vi "Tarea 16.vi"() -> ()   [LabVIEW 2019]
uses:
  Student Material/Student Material/Module 4/Exercises 16/Solutions/CLD 16 state enum.ctl
  Student Material/Student Material/Module 4/Exercises 16/Controls/CLD 16 Status Panel.ctl
  Student Material/Student Material/Module 4/Exercises 16/Controls/CLD 16 Control Panel.ctl
  Student Material/Student Material/Module 4/Exercises 16/Solutions/CLD 16 Data Cluster.ctl
panel:
  out "Error Out":errorcluster
  in  "Error In":errorcluster
  in  "Control Panel Line Two":T1 {"Tons of Peanuts" scale=0.0..10.0}
  in  "Control Panel Line One":T1 {"Tons of Peanuts" scale=0.0..10.0}
  out "Process Control":T2 {"Process Value" format="%#.3g"}
  out "Line One Active":bool
  out "Line Two Active":bool
  in  "Stop Button":bool
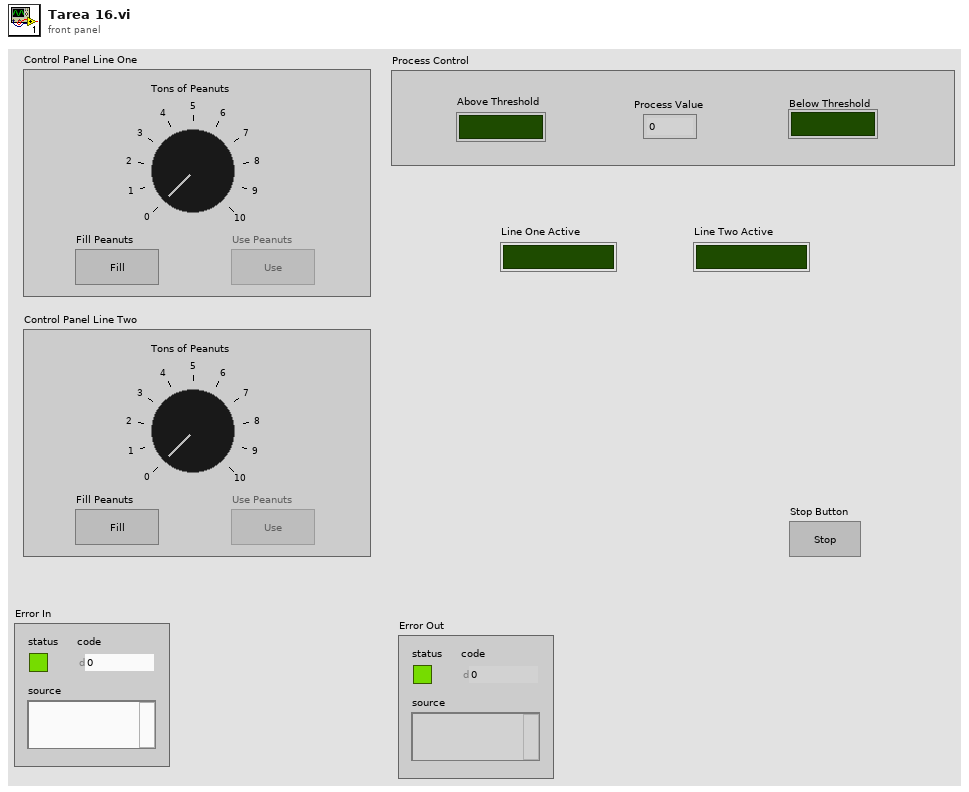
[diagram p1: front panel]
types:
  T1 = typedef "CLD 16 Control Panel.ctl" = cluster{"Tons of Peanuts":i8, "Fill Peanuts":bool, "Use Peanuts":bool}
  T2 = typedef "CLD 16 Status Panel.ctl" = cluster{"Above Threshold":bool, "Below Threshold":bool, "Process Value":dbl}
  T3 = typedef "CLD 16 Data Cluster.ctl" = cluster{"Control Panel Array":T1[], "Status Panel":T2, "Line One":bool, "Line Two":bool, "Stop Button":bool}
  T4 = typedef "CLD 16 state enum.ctl" = enum16{"initialize", "use", "idle"}
  T5 = enum8{"Enabled", "Disabled", "Disabled and Grayed Out"}
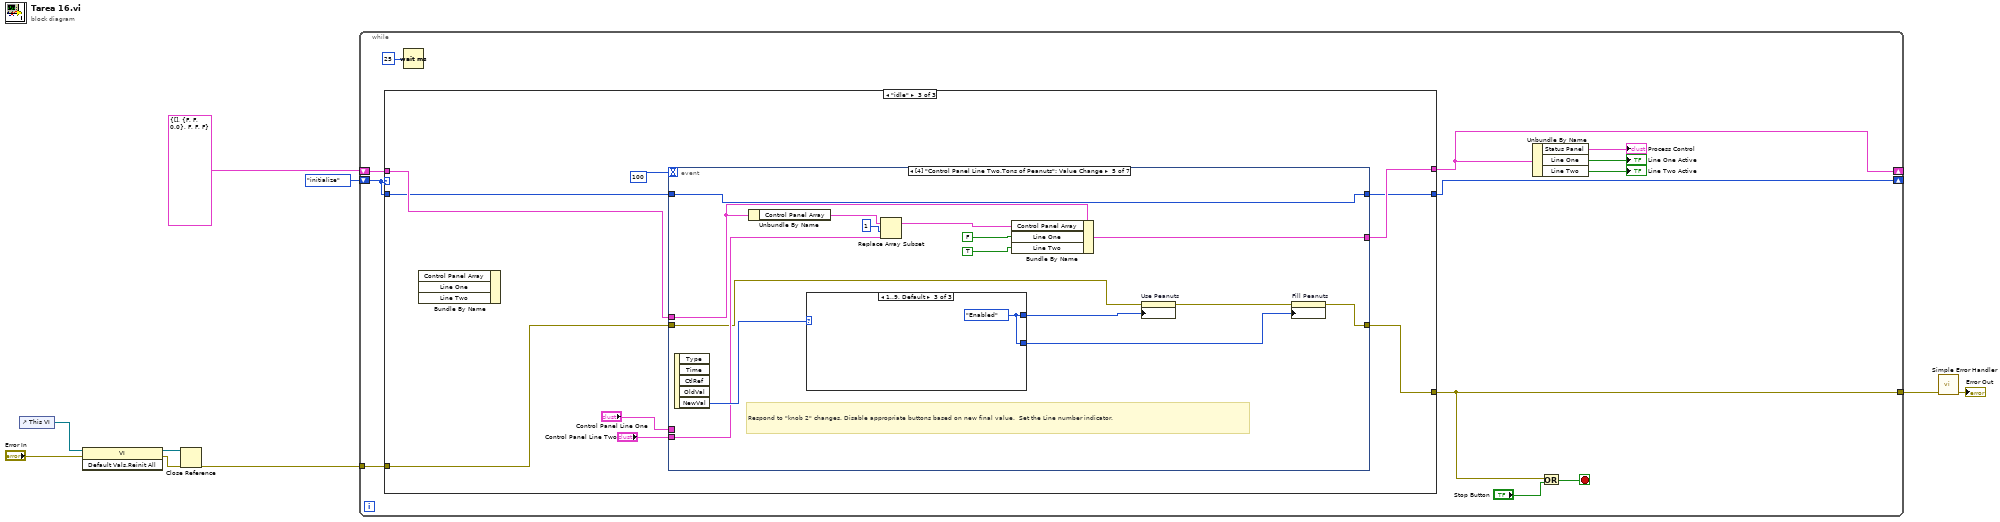
[diagram p0: block diagram]
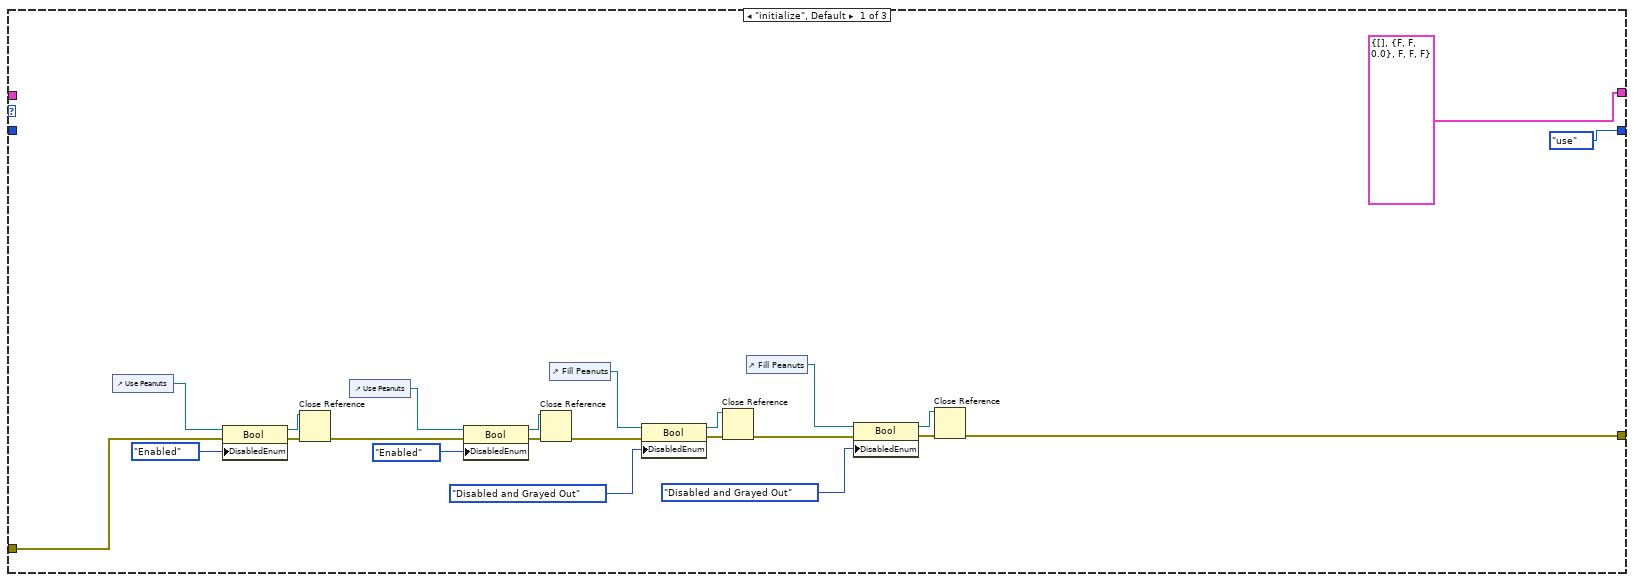
[diagram p2: hidden frame]
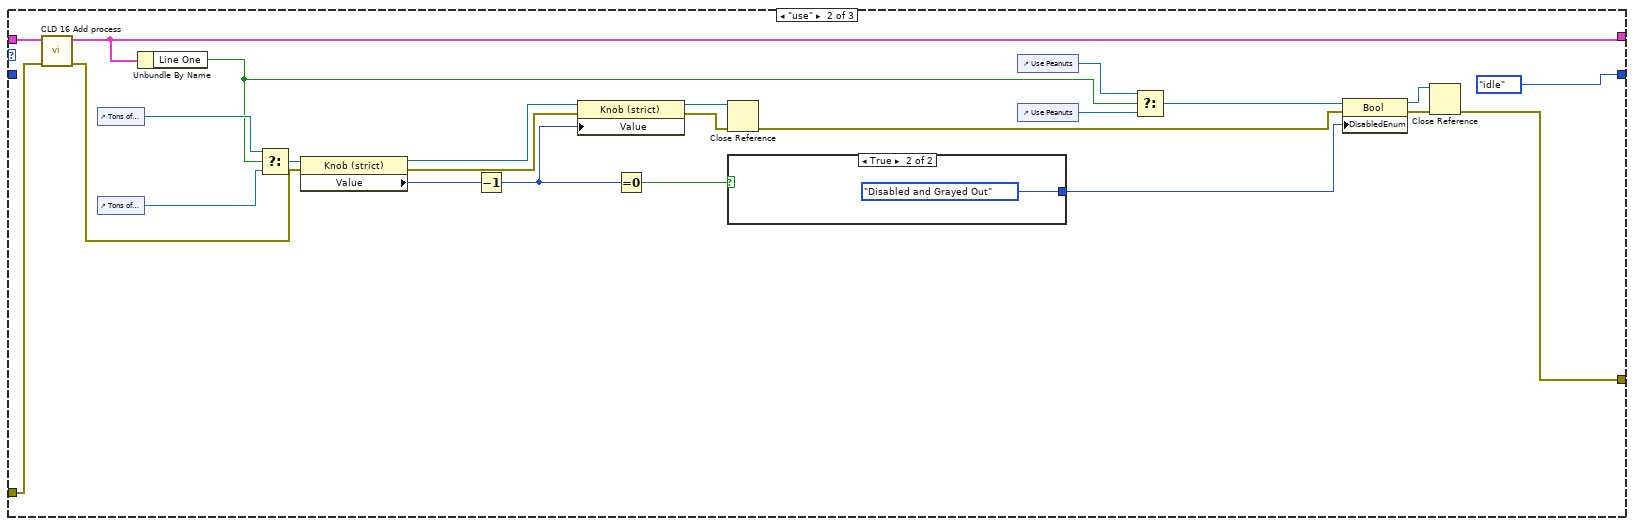
[diagram p3: hidden frame]
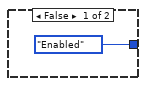
[diagram p4: hidden frame]
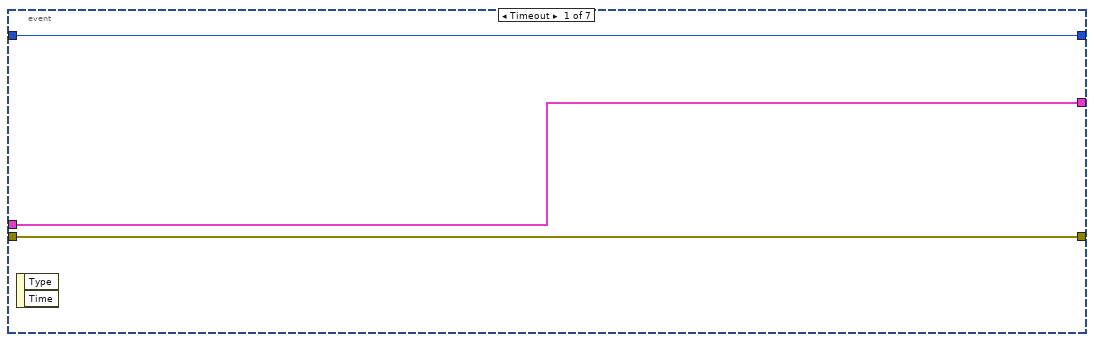
[diagram p5: hidden frame]
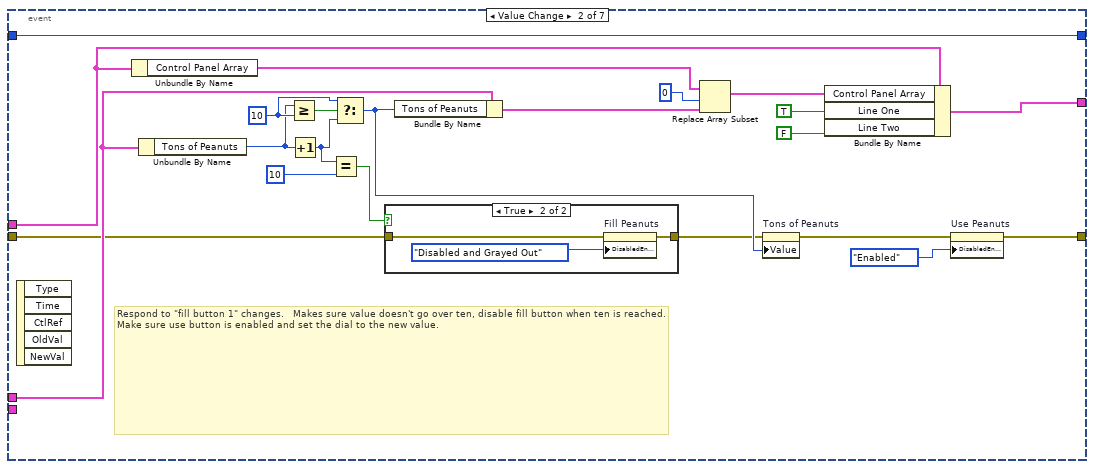
[diagram p6: hidden frame]
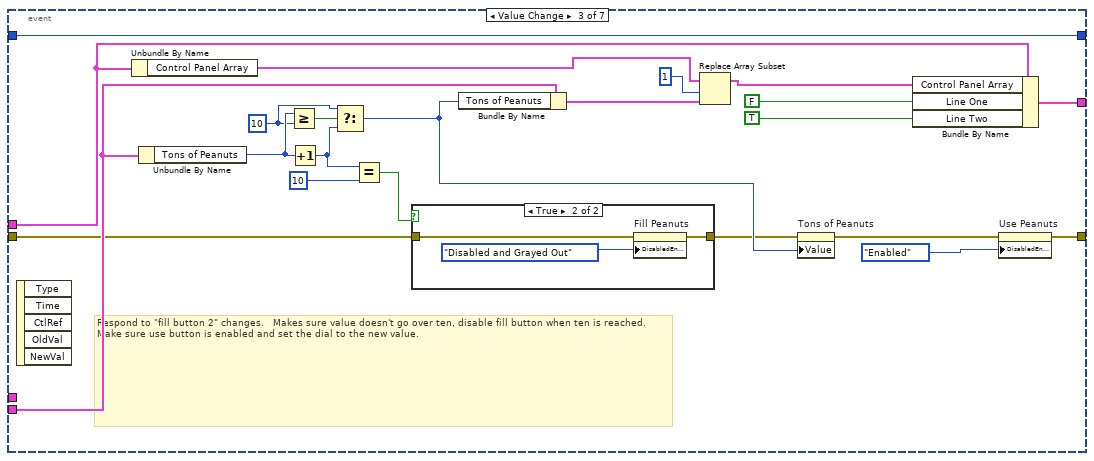
[diagram p8: hidden frame]
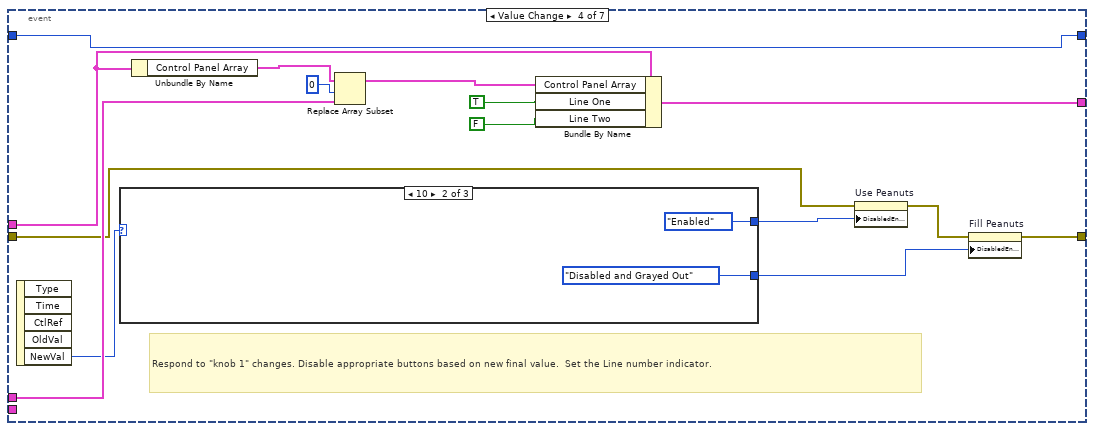
[diagram p10: hidden frame]
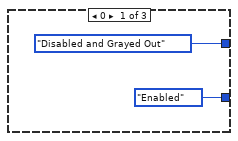
[diagram p11: hidden frame]
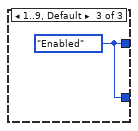
[diagram p12: hidden frame]
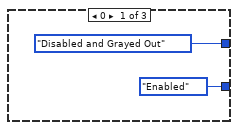
[diagram p13: hidden frame]
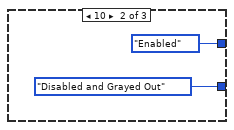
[diagram p14: hidden frame]
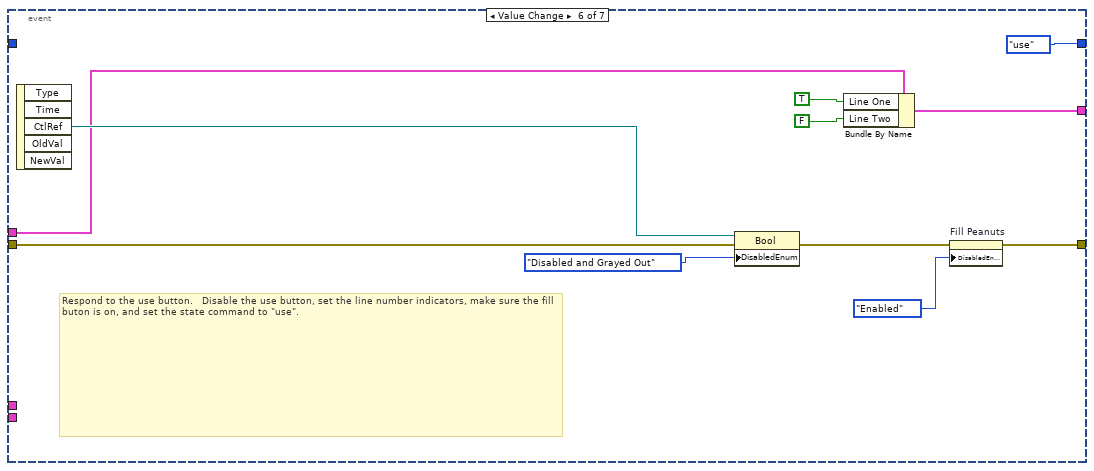
[diagram p15: hidden frame]
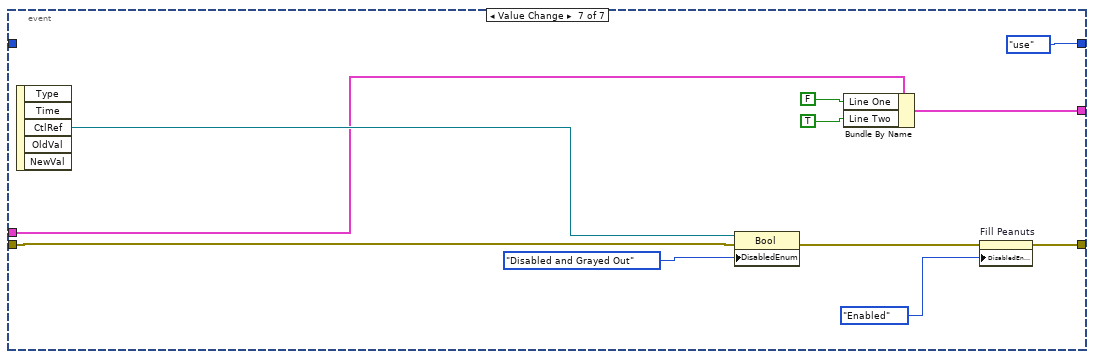
[diagram p16: hidden frame]
diagram:
  n1 = control-ref of="This VI"() -> (w4:refnum<vi>)
  n2 = invoke class="VI" method="Default Vals.Reinit All"(reference=w4, error in="Error In") -> (reference out=w2:refnum<vi>, error out=w5:errorcluster)  [unwired: 1 in, 1 out]
  n3 = Close Reference(reference=w2, error in (no error)=w5) -> (error out=w3:errorcluster)
  n4 = while {
    shift-right: [w20] -> _
    shift-left: CLD_16_state_enum."initialize" ("CLD 16 States") -> [w21]
    shift-right: [w15] -> _
    shift-left: T3 {"Control Panel Array"=[], "Status Panel"={"Above Threshold"=FALSE, "Below Threshold"=FALSE, "Process Value"=0.0}, "Line One"=FALSE, "Line Two"=FALSE, "Stop Button"=FALSE} ("Cluster") -> [w19]
    tunnel: [w10] -> w8
    tunnel: w3 -> [w18]
    stop <- w17 stop-if-true
    n5 = case shown="\"idle\"" w21 {
      tunnel: [CLD_16_state_enum."use" ("CLD 16 States") CLD_16_state_enum."idle" ("CLD 16 States") w74] -> w20
      tunnel: w21 -> [_ _ w75]
      tunnel: w19 -> [_ w68 w79]
      tunnel: [T3 {"Control Panel Array"=[], "Status Panel"={"Above Threshold"=FALSE, "Below Threshold"=FALSE, "Process Value"=0.0}, "Line One"=FALSE, "Line Two"=FALSE, "Stop Button"=FALSE} ("Cluster") w66 w78] -> w15
      tunnel: [w22 w47 w71] -> w10
      tunnel: w18 -> [w29 w46 w72]
      frame "initialize", Default {
        n6 = control-ref of="Use Peanuts"() -> (w30:refnum<vi>)
        n7 = property class="Bool"(reference=w30, error in=w29, "DisabledEnum"=T5."Enabled" ("Disabled")) -> (reference out=w40:refnum<vi>, error out=w42:errorcluster)
        n8 = Close Reference(reference=w40, error in (no error)=w42) -> (error out=w28:errorcluster)
        n9 = control-ref of="Use Peanuts"() -> (w27:refnum<vi>)
        n10 = property class="Bool"(reference=w27, error in=w28, "DisabledEnum"=T5."Enabled" ("Disabled")) -> (reference out=w37:refnum<vi>, error out=w39:errorcluster)
        n11 = Close Reference(reference=w37, error in (no error)=w39) -> (error out=w26:errorcluster)
        n12 = control-ref of="Fill Peanuts"() -> (w25:refnum<vi>)
        n13 = property class="Bool"(reference=w25, error in=w26, "DisabledEnum"=T5."Disabled and Grayed Out" ("Disabled")) -> (reference out=w35:refnum<vi>, error out=w36:errorcluster)
        n14 = Close Reference(reference=w35, error in (no error)=w36) -> (error out=w24:errorcluster)
        n15 = control-ref of="Fill Peanuts"() -> (w23:refnum<vi>)
        n16 = property class="Bool"(reference=w23, error in=w24, "DisabledEnum"=T5."Disabled and Grayed Out" ("Disabled")) -> (reference out=w32:refnum<vi>, error out=w33:errorcluster)
        n17 = Close Reference(reference=w32, error in (no error)=w33) -> (error out=w22:errorcluster)
      }
      frame "use" {
        n18 = call "CLD 16 Add process.vi"("error in (no error)"=w46, "Cluster in"=w68) -> ("error out"=w45:errorcluster, "Cluster out"=w66:T3)  [unwired: 8 in]
        n19 = control-ref of="Tons of Peanuts"() -> (w58:refnum<vi>)
        n20 = control-ref of="Tons of Peanuts"() -> (w59:refnum<vi>)
        n21 = Unbundle By Name(w66) -> ("Line One"=w57:bool)
        n22 = Select(t=w58, s=w57, f=w59) -> (s? t:f=w55:refnum<vi>)
        n23 = property class="Knob (strict)"(reference=w55, error in=w45) -> (reference out=w54:refnum<vi>, error out=w49:errorcluster, "Value"=w56:i8)
        n24 = Decrement(x=w56) -> (x-1=w51:i8)
        n25 = property class="Knob (strict)"(reference=w54, error in=w49, "Value"=w51) -> (reference out=w52:refnum<vi>, error out=w53:errorcluster)
        n26 = Equal To 0?(x=w51) -> (x = 0?=w50:bool)
        n27 = Close Reference(reference=w52, error in (no error)=w53) -> (error out=w48:errorcluster)
        n28 = case shown="True" w50 {
          tunnel: [T5."Enabled" ("Disabled") T5."Disabled and Grayed Out" ("Disabled")] -> w63
          frame False {
          }
          frame True {
          }
        }
        n29 = control-ref of="Use Peanuts"() -> (w65:refnum<vi>)
        n30 = control-ref of="Use Peanuts"() -> (w62:refnum<vi>)
        n31 = Select(t=w65, s=w57, f=w62) -> (s? t:f=w64:refnum<vi>)
        n32 = property class="Bool"(reference=w64, error in=w48, "DisabledEnum"=w63) -> (reference out=w60:refnum<vi>, error out=w61:errorcluster)
        n33 = Close Reference(reference=w60, error in (no error)=w61) -> (error out=w47:errorcluster)
      }
      frame "idle" {
        n34 = Bundle By Name() -> ()  [unwired: 4 in, 1 out]
        n35 = event shown="[4] \"Control Panel Line Two.Tons of Peanuts\": Value Change" {
          selector: _ -> [_ _ _ _ _ _ _]
          dyn-events: _ -> [_ _ _ _ _ _ _]
          timeout: 100 -> [_ _ _ _ _ _ _]
          tunnel: w79 -> [w81 w103 w129 w148 w168 w180 w191]
          tunnel: [w81 w104 w130 w149 w169 w179 w190] -> w78
          tunnel: "Control Panel Line One" -> [_ w96 _ w141 _ _ _]
          tunnel: [w82 w99 w125 w144 w164 CLD_16_state_enum."use" ("CLD 16 States") CLD_16_state_enum."use" ("CLD 16 States")] -> w74
          tunnel: w75 -> [w82 w99 w125 w144 w164 _ _]
          tunnel: "Control Panel Line Two" -> [_ _ w116 _ w159 _ _]
          tunnel: w72 -> [w80 w91 w115 w138 w158 w178 w189]
          tunnel: [w80 w89 w113 w136 w156 w176 w187] -> w71
          event Timeout {
            n36 = event-data() -> ()  [unwired: 1 in, 2 out]
          }
          event Value Change {
            w92 = i8 10 ("x")
            # "Respond to \"fill button 1\" changes.   Makes sure value doesn't go over ten, disable fill button when ten is reached. Make sure use button is enabled and set the dial to the new value."
            n37 = event-data() -> ()  [unwired: 1 in, 5 out]
            n38 = Unbundle By Name(w103) -> ("Control Panel Array"=w102:T1[])
            n39 = Unbundle By Name(w96) -> ("Tons of Peanuts"=w84:i8)
            n40 = Greater Or Equal?(x=w84, y=w92) -> (x >= y?=w87:bool)
            n41 = Increment(x=w84) -> (x+1=w83:i8)
            n42 = Equal?(x=w83, y=i8 10 ("x")) -> (x = y?=w85:bool)
            n43 = Select(t=w92, s=w87, f=w83) -> (s? t:f=w93:i8)
            n44 = case shown="True" w85 {
              tunnel: w91 -> [w105 w108]
              tunnel: [w105 w107] -> w88
              frame False {
              }
              frame True {
                n45 = property on="Fill Peanuts" class="Bool"(error in=w108, "DisabledEnum"=T5."Disabled and Grayed Out" ("Disabled")) -> (error out=w107:errorcluster)  [unwired: 1 in, 1 out]
              }
            }
            n46 = Bundle By Name(cluster=w96, "Tons of Peanuts"=w93) -> (w95:T1)
            n47 = Replace Array Subset(array=w102, new element=w95, index=0) -> (w100:T1[])
            n48 = property on="Tons of Peanuts" class="Knob (strict)"(error in=w88, "Value"=w93) -> (error out=w90:errorcluster)  [unwired: 1 in, 1 out]
            n49 = Bundle By Name(cluster=w103, "Control Panel Array"=w100, "Line One"=TRUE, "Line Two"=FALSE ("Line One")) -> (w104:T3)
            n50 = property on="Use Peanuts" class="Bool"(error in=w90, "DisabledEnum"=T5."Enabled" ("Disabled")) -> (error out=w89:errorcluster)  [unwired: 1 in, 1 out]
          }
          event Value Change {
            w117 = i8 10 ("x")
            # "Respond to \"fill button 2\" changes.   Makes sure value doesn't go over ten, disable fill button when ten is reached. Make sure use button is enabled and set the dial to the new value."
            n51 = event-data() -> ()  [unwired: 1 in, 5 out]
            n52 = Unbundle By Name(w129) -> ("Control Panel Array"=w128:T1[])
            n53 = Unbundle By Name(w116) -> ("Tons of Peanuts"=w118:i8)
            n54 = Greater Or Equal?(x=w118, y=w117) -> (x >= y?=w120:bool)
            n55 = Increment(x=w118) -> (x+1=w111:i8)
            n56 = Select(t=w117, s=w120, f=w111) -> (s? t:f=w119:i8)
            n57 = Equal?(x=w111, y=i8 10 ("x")) -> (x = y?=w109:bool)
            n58 = case shown="True" w109 {
              tunnel: w115 -> [w131 w134]
              tunnel: [w131 w133] -> w110
              frame False {
              }
              frame True {
                n59 = property on="Fill Peanuts" class="Bool"(error in=w134, "DisabledEnum"=T5."Disabled and Grayed Out" ("Disabled")) -> (error out=w133:errorcluster)  [unwired: 1 in, 1 out]
              }
            }
            n60 = Bundle By Name(cluster=w116, "Tons of Peanuts"=w119) -> (w122:T1)
            n61 = Replace Array Subset(array=w128, new element=w122, index=1) -> (w126:T1[])
            n62 = property on="Tons of Peanuts" class="Knob (strict)"(error in=w110, "Value"=w119) -> (error out=w114:errorcluster)  [unwired: 1 in, 1 out]
            n63 = Bundle By Name(cluster=w129, "Control Panel Array"=w126, "Line One"=FALSE, "Line Two"=TRUE ("Line One")) -> (w130:T3)
            n64 = property on="Use Peanuts" class="Bool"(error in=w114, "DisabledEnum"=T5."Enabled" ("Disabled")) -> (error out=w113:errorcluster)  [unwired: 1 in, 1 out]
          }
          event Value Change {
            # "Respond to \"knob 1\" changes. Disable appropriate buttons based on new final value.  Set the Line number indicator."
            n65 = event-data() -> ("NewVal"=w139:i8)  [unwired: 1 in, 4 out]
            n66 = case shown="10" w139 {
              tunnel: [T5."Disabled and Grayed Out" ("Disabled") T5."Enabled" ("Disabled") w154] -> w140
              tunnel: [T5."Enabled" ("Disabled") T5."Disabled and Grayed Out" ("Disabled") w154] -> w135
              frame 0 {
              }
              frame 10 {
              }
              frame 1..9, Default {
                w154 = T5."Enabled" ("Disabled")
              }
            }
            n67 = Unbundle By Name(w148) -> ("Control Panel Array"=w147:T1[])
            n68 = Replace Array Subset(array=w147, new element=w141, index=0) -> (w145:T1[])
            n69 = Bundle By Name(cluster=w148, "Control Panel Array"=w145, "Line One"=TRUE, "Line Two"=FALSE ("Line One")) -> (w149:T3)
            n70 = property on="Use Peanuts" class="Bool"(error in=w138, "DisabledEnum"=w140) -> (error out=w137:errorcluster)  [unwired: 1 in, 1 out]
            n71 = property on="Fill Peanuts" class="Bool"(error in=w137, "DisabledEnum"=w135) -> (error out=w136:errorcluster)  [unwired: 1 in, 1 out]
          }
          event Value Change {
            # "Respond to \"knob 2\" changes. Disable appropriate buttons based on new final value.  Set the Line number indicator."
            n72 = event-data() -> ("NewVal"=w160:i8)  [unwired: 1 in, 4 out]
            n73 = Unbundle By Name(w168) -> ("Control Panel Array"=w167:T1[])
            n74 = case shown="1..9, Default" w160 {
              tunnel: [T5."Disabled and Grayed Out" ("Disabled") T5."Enabled" ("Disabled") w174] -> w161
              tunnel: [T5."Enabled" ("Disabled") T5."Disabled and Grayed Out" ("Disabled") w174] -> w155
              frame 0 {
              }
              frame 10 {
              }
              frame 1..9, Default {
                w174 = T5."Enabled" ("Disabled")
              }
            }
            n75 = Replace Array Subset(array=w167, new element=w159, index=1) -> (w165:T1[])
            n76 = Bundle By Name(cluster=w168, "Control Panel Array"=w165, "Line One"=FALSE, "Line Two"=TRUE ("Line One")) -> (w169:T3)
            n77 = property on="Use Peanuts" class="Bool"(error in=w158, "DisabledEnum"=w161) -> (error out=w157:errorcluster)  [unwired: 1 in, 1 out]
            n78 = property on="Fill Peanuts" class="Bool"(error in=w157, "DisabledEnum"=w155) -> (error out=w156:errorcluster)  [unwired: 1 in, 1 out]
          }
          event Value Change {
            # "Respond to the use button.   Disable the use button, set the line number indicators, make sure the fill buton is on, and set the state command to \"use\"."
            n79 = event-data() -> ("CtlRef"=w184:refnum<vi>)  [unwired: 1 in, 4 out]
            n80 = property class="Bool"(reference=w184, error in=w178, "DisabledEnum"=T5."Disabled and Grayed Out" ("Disabled")) -> (error out=w177:errorcluster)  [unwired: 1 out]
            n81 = Bundle By Name(cluster=w180, "Line One"=TRUE, "Line Two"=FALSE ("Line One")) -> (w179:T3)
            n82 = property on="Fill Peanuts" class="Bool"(error in=w177, "DisabledEnum"=T5."Enabled" ("Disabled")) -> (error out=w176:errorcluster)  [unwired: 1 in, 1 out]
          }
          event Value Change {
            n83 = event-data() -> ("CtlRef"=w195:refnum<vi>)  [unwired: 1 in, 4 out]
            n84 = property class="Bool"(reference=w195, error in=w189, "DisabledEnum"=T5."Disabled and Grayed Out" ("Disabled")) -> (error out=w188:errorcluster)  [unwired: 1 out]
            n85 = Bundle By Name(cluster=w191, "Line One"=FALSE, "Line Two"=TRUE ("Line One")) -> (w190:T3)
            n86 = property on="Fill Peanuts" class="Bool"(error in=w188, "DisabledEnum"=T5."Enabled" ("Disabled")) -> (error out=w187:errorcluster)  [unwired: 1 in, 1 out]
          }
        }
      }
    }
    n87 = Wait (ms)(milliseconds to wait=u32 25) -> ()  [unwired: 1 out]
    n88 = Unbundle By Name(w15) -> ("Status Panel"=→"Process Control":T2, "Line One"=→"Line One Active":bool, "Line Two"=→"Line Two Active":bool)
    n89 = Or(x=w10, y="Stop Button") -> (x .or. y?=w17:bool)
  }
  n90 = call <vilib>:"Simple Error Handler.vi"("error in (no error)"=w8) -> ("error out"=→"Error Out":errorcluster)  [unwired: 4 in, 4 out]
